vi "getCapacitance.vi"(8 "error in (no error)":errorcluster, 9 "Channel":i32, 11 "Instrument.CBridge in":refnum<class "Instrument.CBridge.lvclass">) -> (0 "error out":errorcluster, 2 "Capacitance (pF)":dbl, 3 "Instrument.CBridge out":refnum<class "Instrument.CBridge.lvclass">)   [LabVIEW 2019, in "Instrument.CBridge.lvclass"]
uses:
  Instrument.CBridge.lvclass
  Instrument/Instrument.lvclass
  25fccf32-2e48-4427-8a98-5ba8f6b1c5e8.vi
  C:/Users/patrick/Documents/GitHub/Instrument-Framework/lvsrc/Instrument/Instrument.lvclass
  C:/Program Files (x86)/National Instruments/LabVIEW 2019/vi.lib/JKI/JKI SMO/SMO/SMO.lvclass
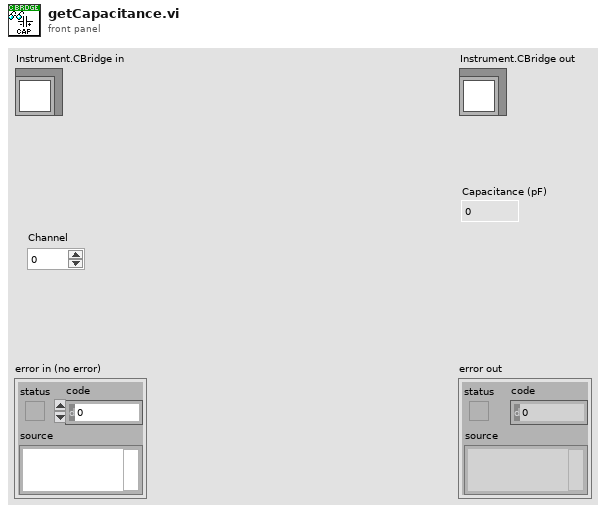
[diagram p1: front panel]
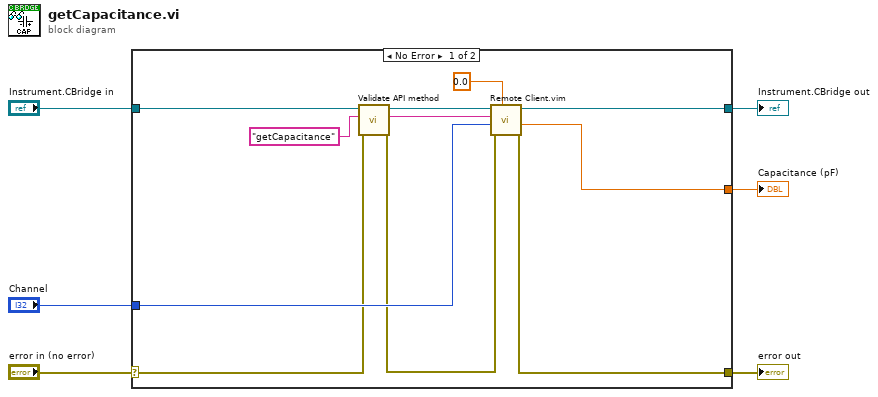
[diagram p0: block diagram]
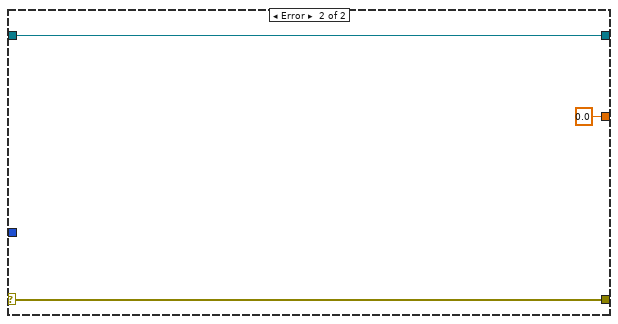
[diagram p2: hidden frame]
diagram:
  n1 = case shown="No Error" "error in (no error)" {
    selector: "error in (no error)" -> [w8 w20]
    tunnel: [w12 w20] -> w5
    tunnel: [w11 w19] -> w3
    tunnel: "Instrument.CBridge in" -> [w13 w19]
    tunnel: [w10 0.0 ("Data out")] -> w2
    tunnel: "Channel" -> [w9 _]
    frame No Error {
      n2 = call "Validate API method.vi"("error in (no error)"=w8, "Command in"="getCapacitance" ("error message (\"\")"), "Instrument in"=w13) -> ("error out"=w7:errorcluster, "command out"=w15:string, "Instrument out"=w14:refnum<class "Instrument.CBridge.lvclass">)  [unwired: 6 in]
      n3 = call "Remote Client.vim"("Command out"=w15, "Data Out type"=0.0, "error in (no error)"=w7, "Data in"=w9, "Instrument in"=w14) -> ("error out"=w12:errorcluster, "Data out"=w10:dbl, "Instrument out"=w11:refnum<class "Instrument.CBridge.lvclass">)  [unwired: 4 in]
    }
    frame Error {
    }
  }
  "error out" <- w5
  "Instrument.CBridge out" <- w3
  "Capacitance (pF)" <- w2
